vi "Set Func.vi"(8 "error in (no error)":errorcluster caption="entrée d'erreur (pas d'erreur)", 10 "Func":string, 11 "Parsing Data RADIO_ERP1_A5_02_05 en entrée":refnum<class "Parsing Data RADIO_ERP1_A5_H.lvclass">) -> (0 "error out":errorcluster caption="sortie d'erreur", 3 "Parsing Data RADIO_ERP1_A5_02_05 en sortie":refnum<class "Parsing Data RADIO_ERP1_A5_H.lvclass">)   [LabVIEW 2020, in "Library Instrument & Equipement.lvlib" / "Library UART.lvlib" / "Parsing Data RADIO_ERP1_A5_H.lvclass"]
uses:
  Parsing Data RADIO_ERP1_A5_H.lvclass
  Parsing Data RADIO_ERP1_A5_H.lvclass/Parsing Data RADIO_ERP1_A5_H.ctl
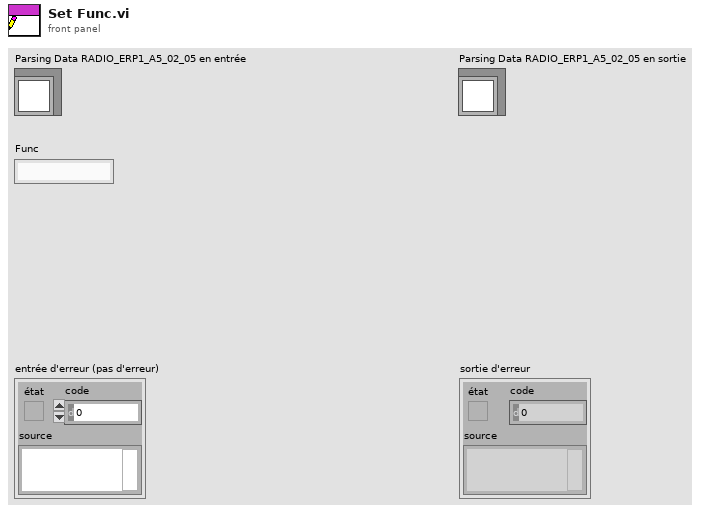
[diagram p1: front panel]
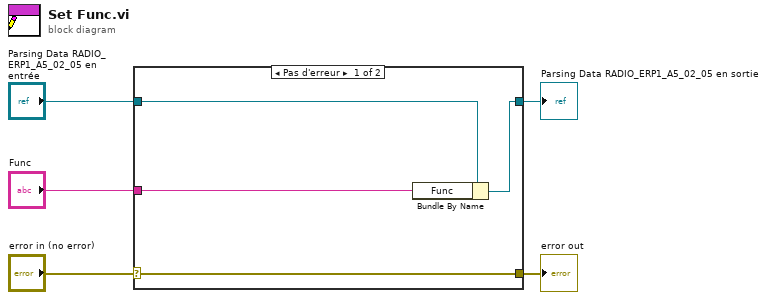
[diagram p0: block diagram]
diagram:
  n1 = case shown="Pas d'erreur" "error in (no error)" {
    selector: "error in (no error)" -> [w9 w10]
    tunnel: [w9 w10] -> w4
    tunnel: [w7 w11] -> w2
    tunnel: "Parsing Data RADIO_ERP1_A5_02_05 en entrée" -> [w8 w11]
    tunnel: "Func" -> [w6 _]
    frame No Error {
      n2 = Bundle By Name(cluster=w8, "Func"=w6) -> (w7:refnum<class "Parsing Data RADIO_ERP1_A5_H.lvclass">)
    }
    frame Error {
    }
  }
  "error out" <- w4
  "Parsing Data RADIO_ERP1_A5_02_05 en sortie" <- w2
